vi "Constructor.vi"(10 "Beverage":refnum<class "Beverage.lvclass">, 11 "Mocha in":refnum<class "Mocha.lvclass">) -> (3 "Mocha out":refnum<class "Mocha.lvclass">)   [LabVIEW 2011, in "Mocha.lvclass"]
uses:
  Mocha.lvclass
  Beverage/Beverage.lvclass
  Mocha.lvclass/Mocha.ctl
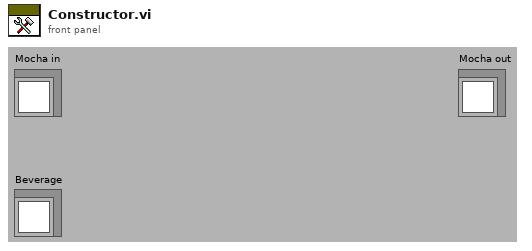
[diagram p1: front panel]
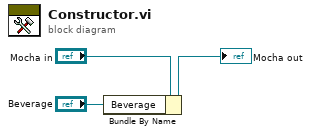
[diagram p0: block diagram]
diagram:
  n1 = Bundle By Name(cluster="Mocha in", "Beverage"="Beverage") -> (→"Mocha out":refnum<class "Mocha.lvclass">)
